vi "Clear Scan Time Out - 複製 (2).vi"(6 "ESP32 error in (no error) 2":errorcluster, 7 "ESP32 ref":refnum<visa-resource-name>="COM4", 8 "DMM error in (no error)":errorcluster, 11 "VISA Refnum in":refnum<visa-resource-name>) -> (0 "DMM error out":errorcluster, 1 "error?":bool, 2 "Time out count":i32, 3 "VISA Refnum out":refnum<visa-resource-name>, 4 "DMM error out":errorcluster, 5 "ESP32 ref out":refnum<visa-resource-name>)   [LabVIEW 2023]
uses:
  <vilib>/Utility/error.llb/DialogType.ctl
panel:
  out "Measurements 3":dbl[](array[numeric])
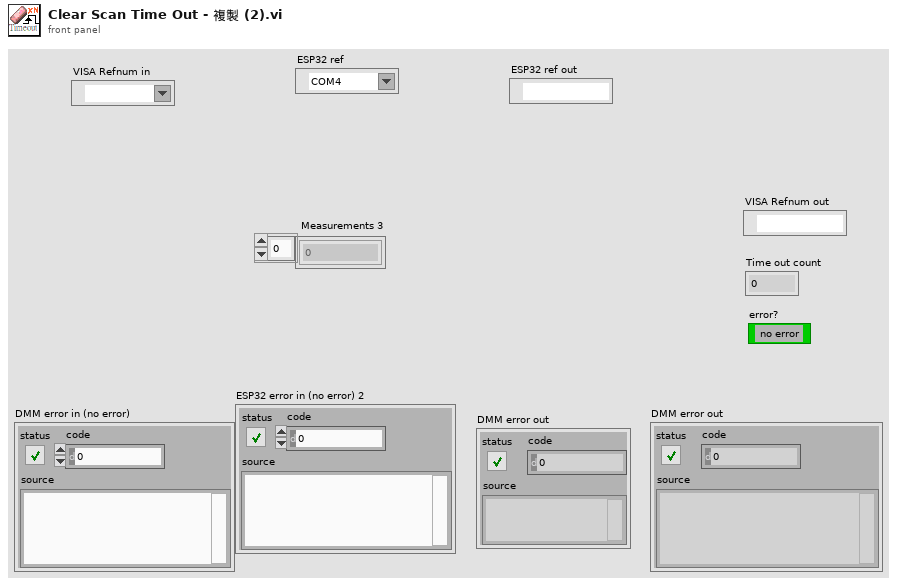
[diagram p1: front panel]
types:
  T1 = typedef "DialogType.ctl" = u16
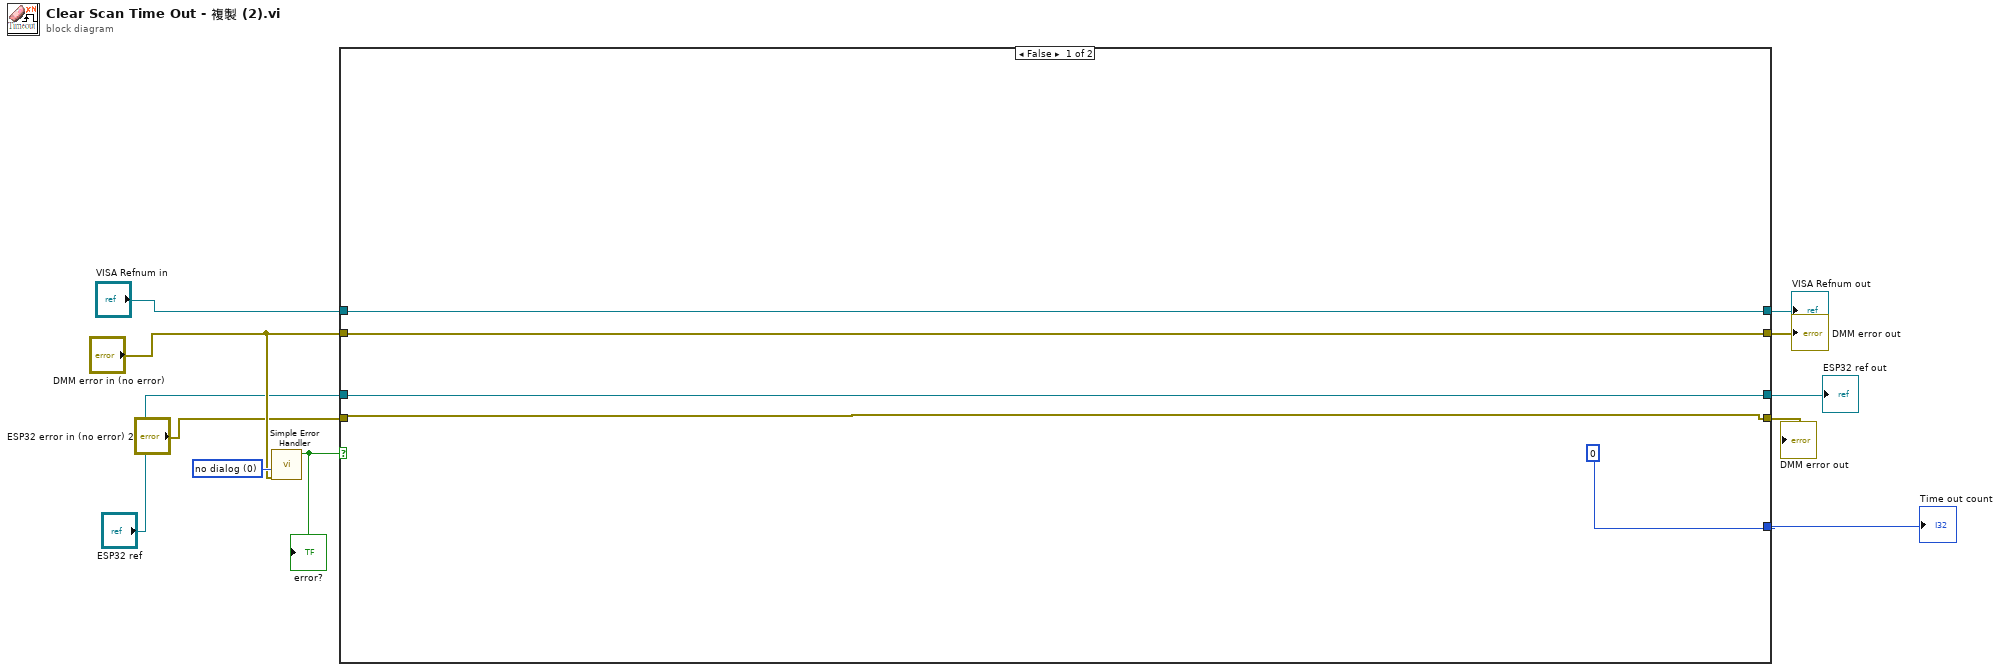
[diagram p0: block diagram]
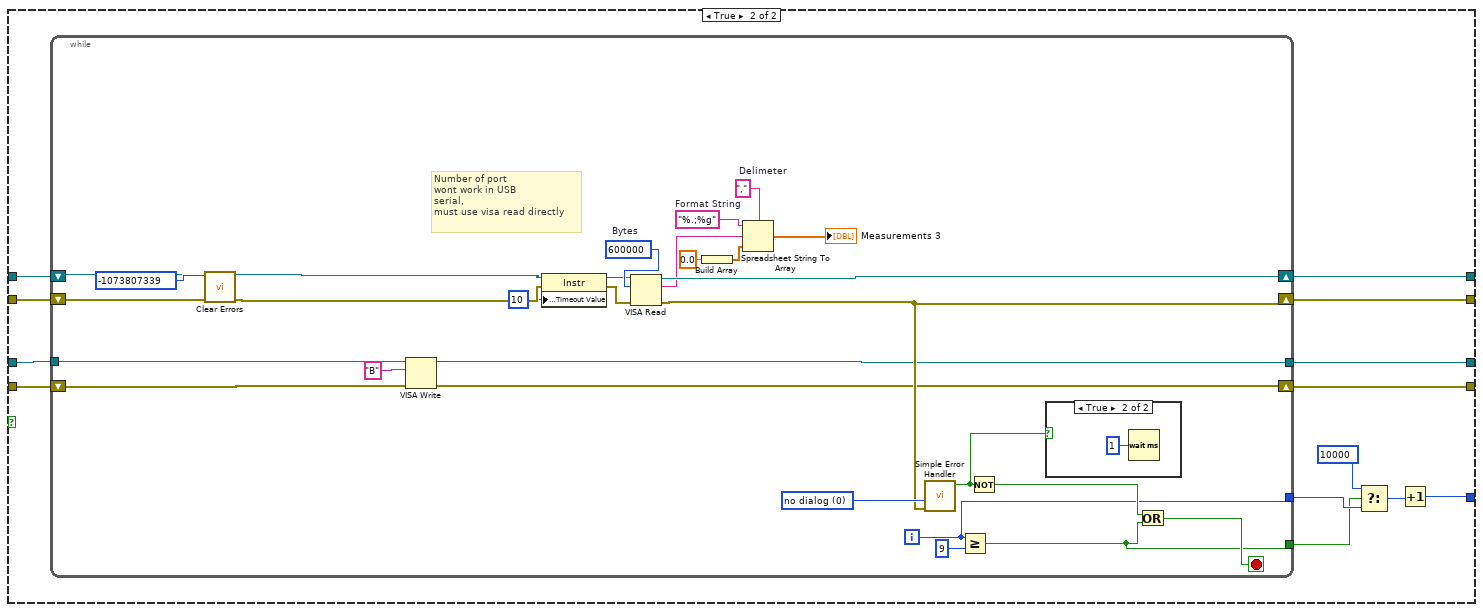
[diagram p2: hidden frame]
diagram:
  w8 = T1 0 items=["no dialog", "OK message", "continue or stop message", "OK message + warnings", "continue/stop + warnings"] ("type of dialog (OK msg:1)")
  n1 = call <vilib>:"Simple Error Handler.vi"("type of dialog (OK msg:1)"=w8, "error in (no error)"="DMM error in (no error)") -> ("error?"=w6:bool)  [unwired: 3 in, 4 out]
  "error?" <- w6
  n2 = case shown="False" w6 {
    tunnel: [w16 w29] -> w11
    tunnel: "DMM error in (no error)" -> [w15 w28]
    tunnel: "VISA Refnum in" -> [w16 w27]
    tunnel: [w15 w26] -> w9
    tunnel: [0 w25] -> w5
    tunnel: "ESP32 ref" -> [w13 w20]
    tunnel: [w13 w19] -> w3
    tunnel: "ESP32 error in (no error) 2" -> [w12 w18]
    tunnel: [w12 w17] -> w1
    frame False {
    }
    frame True {
      n3 = while {
        shift-right: [w52] -> w26
        shift-left: w28 -> [w55]
        shift-right: [w57] -> w29
        shift-left: w27 -> [w34]
        tunnel: [w48] -> w23
        tunnel: [w47] -> w22
        tunnel: w20 -> [w33]
        tunnel: [w32] -> w19
        shift-right: [w30] -> w17
        shift-left: w18 -> [w31]
        i -> [w48]
        stop <- w49 stop-if-true
        w43 = ","  # Delimeter
        w44 = "%.;%g"  # Format String
        w38 = u32 600000  # Bytes
        w53 = T1 0 items=["no dialog", "OK message", "continue or stop message", "OK message + warnings", "continue/stop + warnings"] ("type of dialog (OK msg:1)")
        # "Number of port\nwont work in USB \nserial,\nmust use visa read directly"
        n4 = call <vilib>:"Clear Errors.vi"("error in (no error)"=w55, "specific error code to clear (0: all)"=-1073807339 ("code out")) -> ("error out"=w54:errorcluster)  [unwired: 4 in, 1 out]
        n5 = VISA Write(VISA resource name=w33, write buffer="B", error in (no error)=w31) -> (VISA resource name out=w32:refnum<visa-resource-name>, error out=w30:errorcluster)  [unwired: 1 out]
        n6 = property class="Instr"(reference=w34, error in=w54, "General Settings:Timeout Value"=u32 10) -> (reference out=w37:refnum<visa-resource-name>, error out=w36:errorcluster)
        n7 = VISA Read(VISA resource name=w37, byte count=w38, error in (no error)=w36) -> (VISA resource name out=w57:refnum<visa-resource-name>, read buffer=w39:string, error out=w52:errorcluster)  [unwired: 1 out]
        n8 = Build Array(0.0) -> (w41:dbl[])
        n9 = Spreadsheet String To Array(delimiter (Tab)=w43, format string=w44, spreadsheet string=w39, array type (2D Dbl)=w41) -> (array=→"Measurements 3":dbl[])
        n10 = call <vilib>:"Simple Error Handler.vi"("type of dialog (OK msg:1)"=w53, "error in (no error)"=w52) -> ("error?"=w46:bool)  [unwired: 3 in, 4 out]
        n11 = Greater Or Equal?(x=w48, y=9) -> (x >= y?=w47:bool)
        n12 = Not(x=w46) -> (.not. x?=w50:bool)
        n13 = case shown="True" w46 {
          frame False {
          }
          frame True {
            n14 = Wait (ms)(milliseconds to wait=u32 1) -> ()  [unwired: 1 out]
          }
        }
        n15 = Or(x=w50, y=w47) -> (x .or. y?=w49:bool)
      }
      n16 = Select(t=10000, s=w22, f=w23) -> (s? t:f=w24:i32)
      n17 = Increment(x=w24) -> (x+1=w25:i32)
    }
  }
  "DMM error out" <- w9
  "VISA Refnum out" <- w11
  "Time out count" <- w5
  "ESP32 ref out" <- w3
  "DMM error out" <- w1
